vi "ExSubCloseMultCamPulser.vi"(1 "error in (no error)":errorcluster, 2 "Handles In":T1) -> (0 "error out":errorcluster)   [LabVIEW 2010]
panel:
  # "ExSubCloseMultCamPulser:\nCloses the multiple camera/ptg experiment."
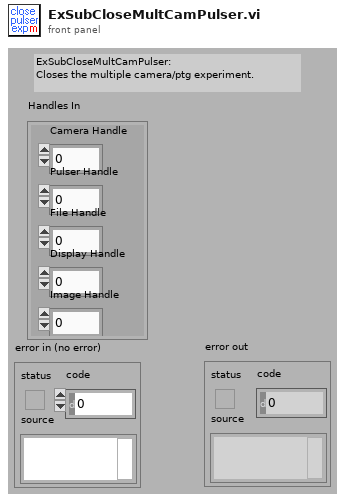
[diagram p1: front panel]
types:
  T1 = cluster{"Camera Handle":u32, "Pulser Handle":u32, "File Handle":u32, "Display Handle":u32, "Image Handle":u32}
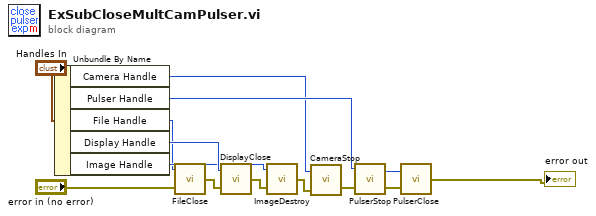
[diagram p0: block diagram]
diagram:
  n1 = Unbundle By Name("Handles In") -> ("Camera Handle"=w2:u32, "Pulser Handle"=w5:u32, "File Handle"=w6:u32, "Display Handle"=w8:u32, "Image Handle"=w7:u32)
  n2 = call <userlib>:"FileClose.vi"("error in"="error in (no error)", "File Handle"=w6) -> ("error out"=w10:errorcluster)
  n3 = call <userlib>:"DisplayClose.vi"("error in"=w10, "Display Handle"=w8) -> ("error out"=w14:errorcluster)
  n4 = call <userlib>:"ImageDestroy.vi"("error in"=w14, "Data handle"=w7) -> ("error out"=w4:errorcluster)
  n5 = call <userlib>:"CameraStop.vi"("error in"=w4, "Camera Handle"=w2) -> ("error out"=w3:errorcluster)  [unwired: 1 out]
  n6 = call <userlib>:"PulserStop.vi"("error in"=w3, "Pulser Handle"=w5) -> ("error out"=w13:errorcluster, "Pulser Handle"=w12:u32)
  n7 = call <userlib>:"PulserClose.vi"("error in (no error)"=w13, "Pulser Handle"=w12) -> ("error out"=→"error out":errorcluster)
